vi "VICI仪器串口通讯.vi"(3 "输入指令":string, 4 "baud rate (9600)":u32=9600, 5 "VISA resource name":refnum<visa-resource-name>="COM3") -> (0 "错误输出":errorcluster, 1 "read buffer":string, 2 "子字符串;substring":string)   [LabVIEW 2016]
uses:
  <vilib>/Instr/_visa.llb/VISA Configure Serial Port (Instr).vi
panel:
  out "输入的字符串":string
  out "返回数 2":u32
  out "返回数":u32
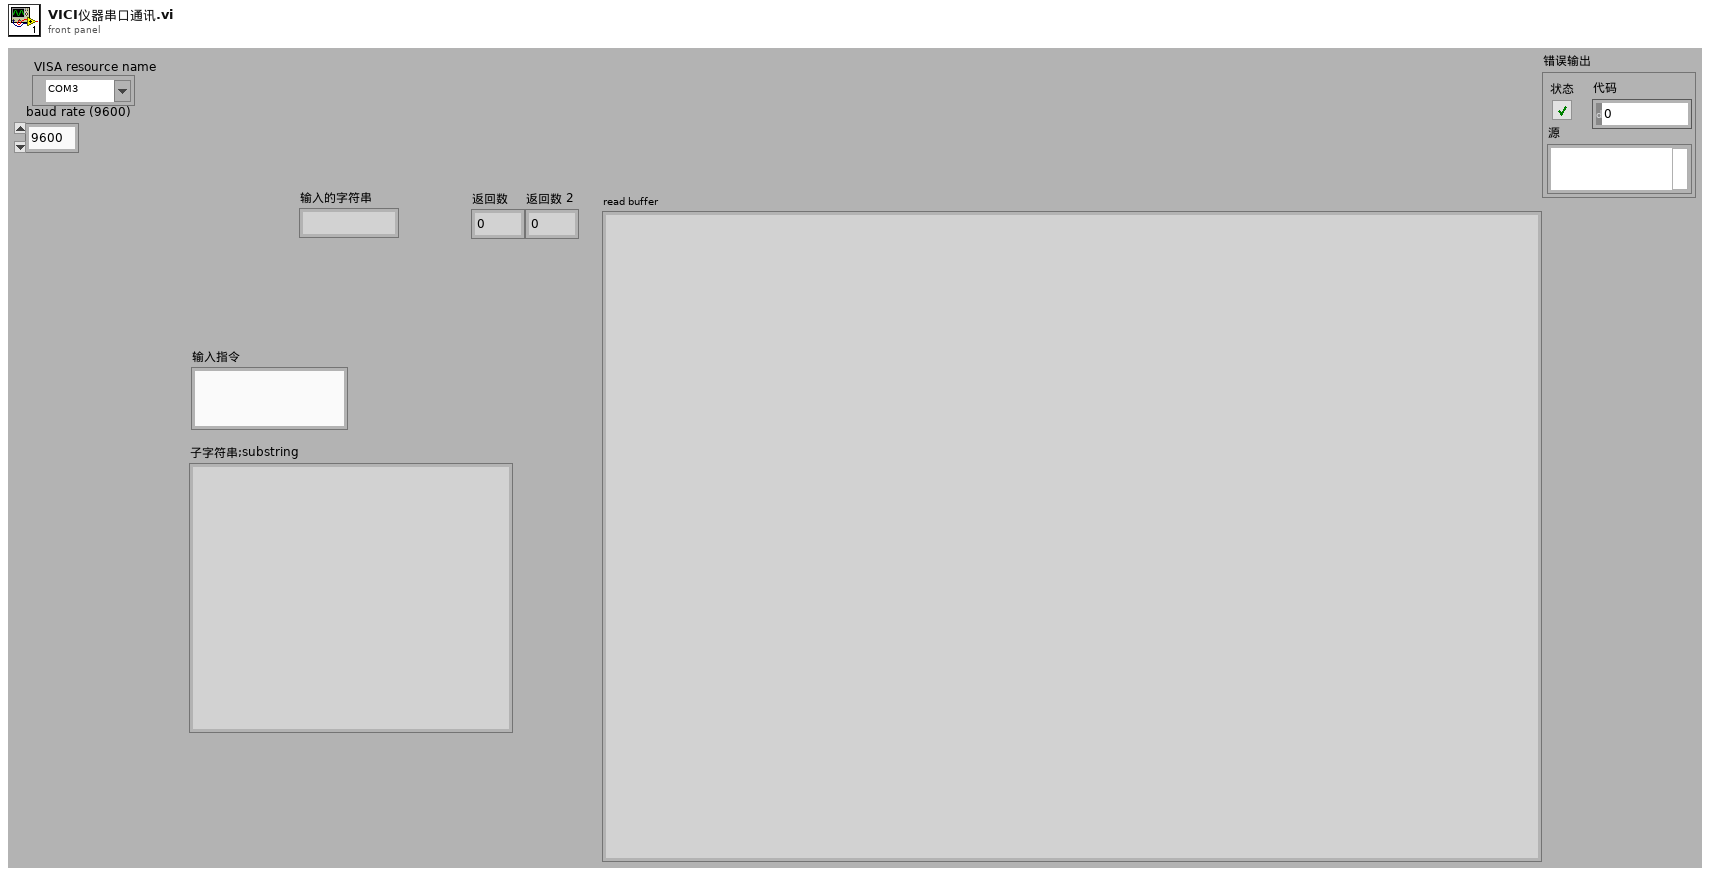
[diagram p1: front panel]
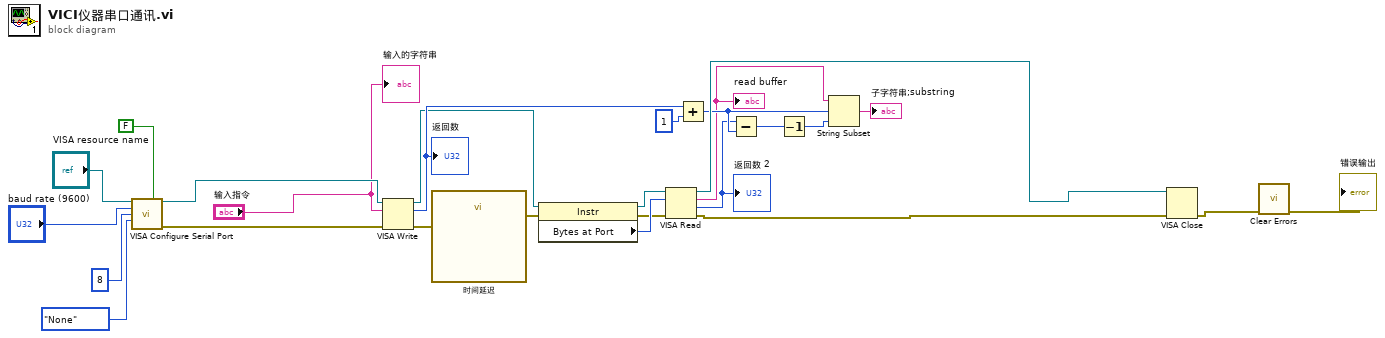
[diagram p0: block diagram]
diagram:
  n1 = call-poly "VISA Configure Serial Port"("VISA resource name"="VISA resource name", "Enable Termination\nChar (T)"=FALSE ("Enable Termination\nChar (T)"), "baud rate (9600)"="baud rate (9600)", "data bits (8)"=u16 8, "parity (0:none)"=enum16{"None", "Odd", "Even", "Mark", "Space"}."None") -> ("VISA resource name out"=w23:refnum<visa-resource-name>, "error out"=w22:errorcluster)  [unwired: 9 in]
  n2 = VISA Write(VISA resource name=w23, write buffer="输入指令", error in (no error)=w22) -> (VISA resource name out=w4:refnum<visa-resource-name>, return count=w9:u32, error out=w17:errorcluster)
  "返回数" <- w9
  n3 = call "时间延迟"("error in (no error)"=w17) -> ("error out"=w16:errorcluster)  [unwired: 10 in]
  n4 = property class="Instr"(reference=w4, error in=w16) -> (reference out=w13:refnum<visa-resource-name>, error out=w14:errorcluster, "Bytes at Port"=w15:u32)
  n5 = VISA Read(VISA resource name=w13, byte count=w15, error in (no error)=w14) -> (VISA resource name out=w20:refnum<visa-resource-name>, read buffer=w8:string, return count=w7:u32, error out=w21:errorcluster)
  "read buffer" <- w8
  "返回数 2" <- w7
  n6 = Add(x=w9, y=1 ("偏移量(0)")) -> (x+y=w11:u32)
  n7 = Subtract(x=w7, y=w11) -> (x-y=w5:u32)
  n8 = Decrement(x=w5) -> (x-1=w6:u32)
  n9 = String Subset(string=w8, offset (0)=w11, length (rest)=w6) -> (substring=→"子字符串;substring":string)
  n10 = VISA Close(VISA resource name=w20, error in (no error)=w21) -> (error out=w19:errorcluster)
  n11 = call <vilib>:"Clear Errors.vi"("error in (no error)"=w19) -> ("error out"=→"错误输出":errorcluster)  [unwired: 5 in, 1 out]
  "输入的字符串" <- "输入指令"
